vi "digitally_ros.vi"() -> ()   [LabVIEW 2019]
uses:
  <vilib>/addons/eal4LabVIEW/ApiLib/Connection control/ealApiConnect_string.vi
  <vilib>/addons/eal4LabVIEW/eal4LabVIEW.lvlib
panel:
  out "appended array":bool[](array[boolean])
  out "In Range? (1)":bool
  out "In Range? (2)":bool
  out "In Range? (3)":bool
  in  "condition 6":i32(ring) items=["AXIS_CONDITION_ACTIVE"=0, "AXIS_CONDITION_PARKING"=1, "AXIS_CONDITION_DEACTIVATED"=2, "AXIS_CONDITION_ACTIVE_DECOUPLED"=4, "AXIS_CONDITION_PARKING_DECOUPLED"=5, "AXIS_CONDITION_DEACTIVATED_DECOUPLED"=6, "AXIS_CONDITION_ACTIVE_PARAMETERIZATION"=8, "AXIS_CONDITION_PARKING_PARAMETERIZATION"=9, "AXIS_CONDITION_DEACTIVATED_PARAMETERIZATION"=10, "AXIS_CONDITION_ACTIVE_DECOUPLED_PARAMETERIZATION"=12, "AXIS_CONDITION_PARKING_DECOUPLED_PARAMETERIZATION"=13, "AXIS_CONDITION_DEACTIVATED_DECOUPLED_PARAMETERIZATION"=14]
  in  "slave index 6":i32
  in  "condition 5":i32(ring) items=["AXIS_CONDITION_ACTIVE"=0, "AXIS_CONDITION_PARKING"=1, "AXIS_CONDITION_DEACTIVATED"=2, "AXIS_CONDITION_ACTIVE_DECOUPLED"=4, "AXIS_CONDITION_PARKING_DECOUPLED"=5, "AXIS_CONDITION_DEACTIVATED_DECOUPLED"=6, "AXIS_CONDITION_ACTIVE_PARAMETERIZATION"=8, "AXIS_CONDITION_PARKING_PARAMETERIZATION"=9, "AXIS_CONDITION_DEACTIVATED_PARAMETERIZATION"=10, "AXIS_CONDITION_ACTIVE_DECOUPLED_PARAMETERIZATION"=12, "AXIS_CONDITION_PARKING_DECOUPLED_PARAMETERIZATION"=13, "AXIS_CONDITION_DEACTIVATED_DECOUPLED_PARAMETERIZATION"=14]
  in  "slave index 5":i32
  in  "condition 4":i32(ring) items=["AXIS_CONDITION_ACTIVE"=0, "AXIS_CONDITION_PARKING"=1, "AXIS_CONDITION_DEACTIVATED"=2, "AXIS_CONDITION_ACTIVE_DECOUPLED"=4, "AXIS_CONDITION_PARKING_DECOUPLED"=5, "AXIS_CONDITION_DEACTIVATED_DECOUPLED"=6, "AXIS_CONDITION_ACTIVE_PARAMETERIZATION"=8, "AXIS_CONDITION_PARKING_PARAMETERIZATION"=9, "AXIS_CONDITION_DEACTIVATED_PARAMETERIZATION"=10, "AXIS_CONDITION_ACTIVE_DECOUPLED_PARAMETERIZATION"=12, "AXIS_CONDITION_PARKING_DECOUPLED_PARAMETERIZATION"=13, "AXIS_CONDITION_DEACTIVATED_DECOUPLED_PARAMETERIZATION"=14]
  in  "slave index 4":i32
  out "RPM Motor 1":dbl
  out "RPM Motor 2":dbl
  out "RPM Motor 3":dbl
  in  "stop":bool
  out "return value":dbl[](array[numeric])
  out "Iteration counter":i32
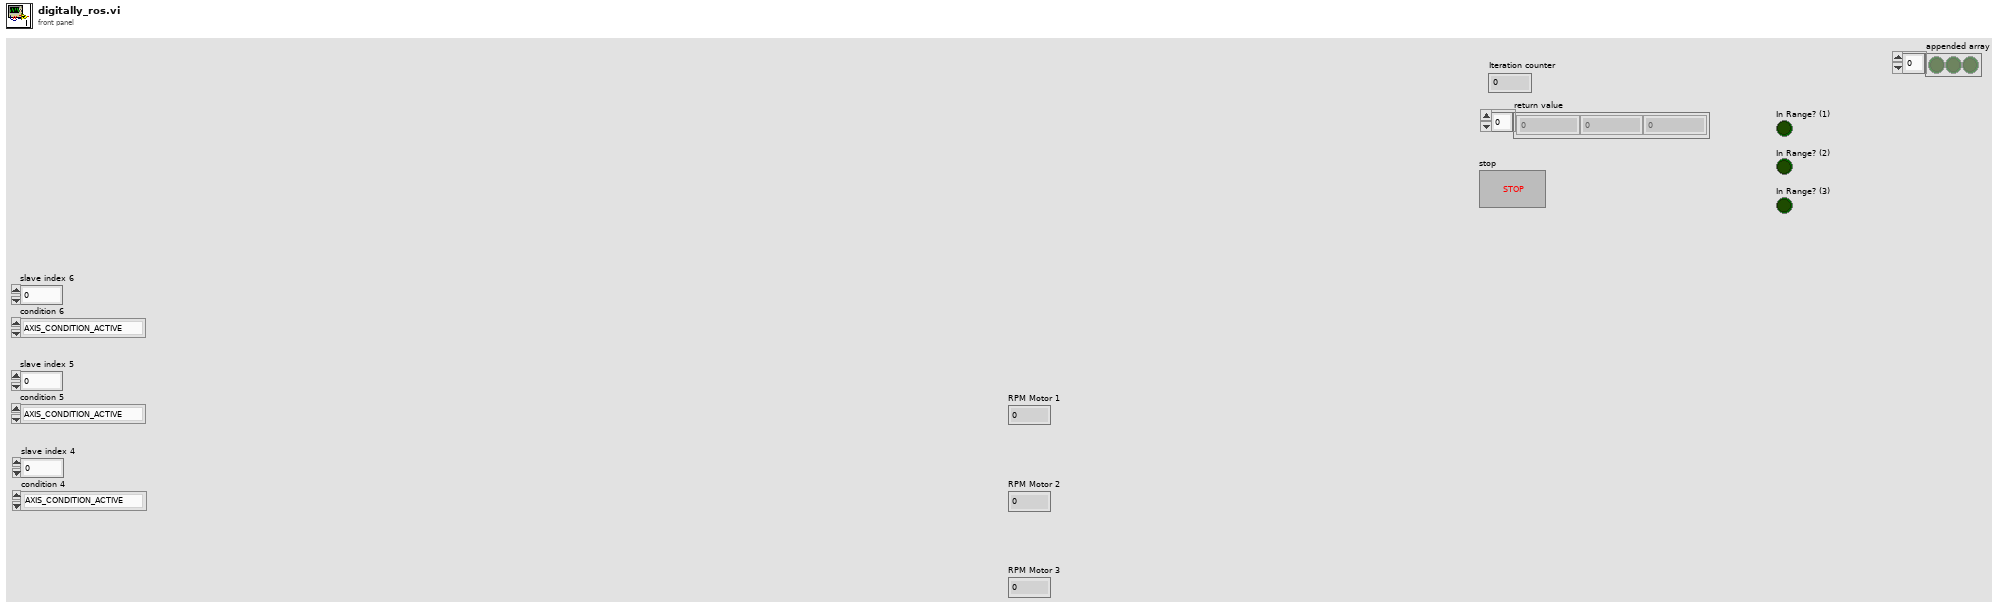
[diagram p1: front panel]
types:
  T1 = cluster{"Velocity":dbl, "Acceleration":dbl, "Deceleration":dbl, "Jerk":dbl}
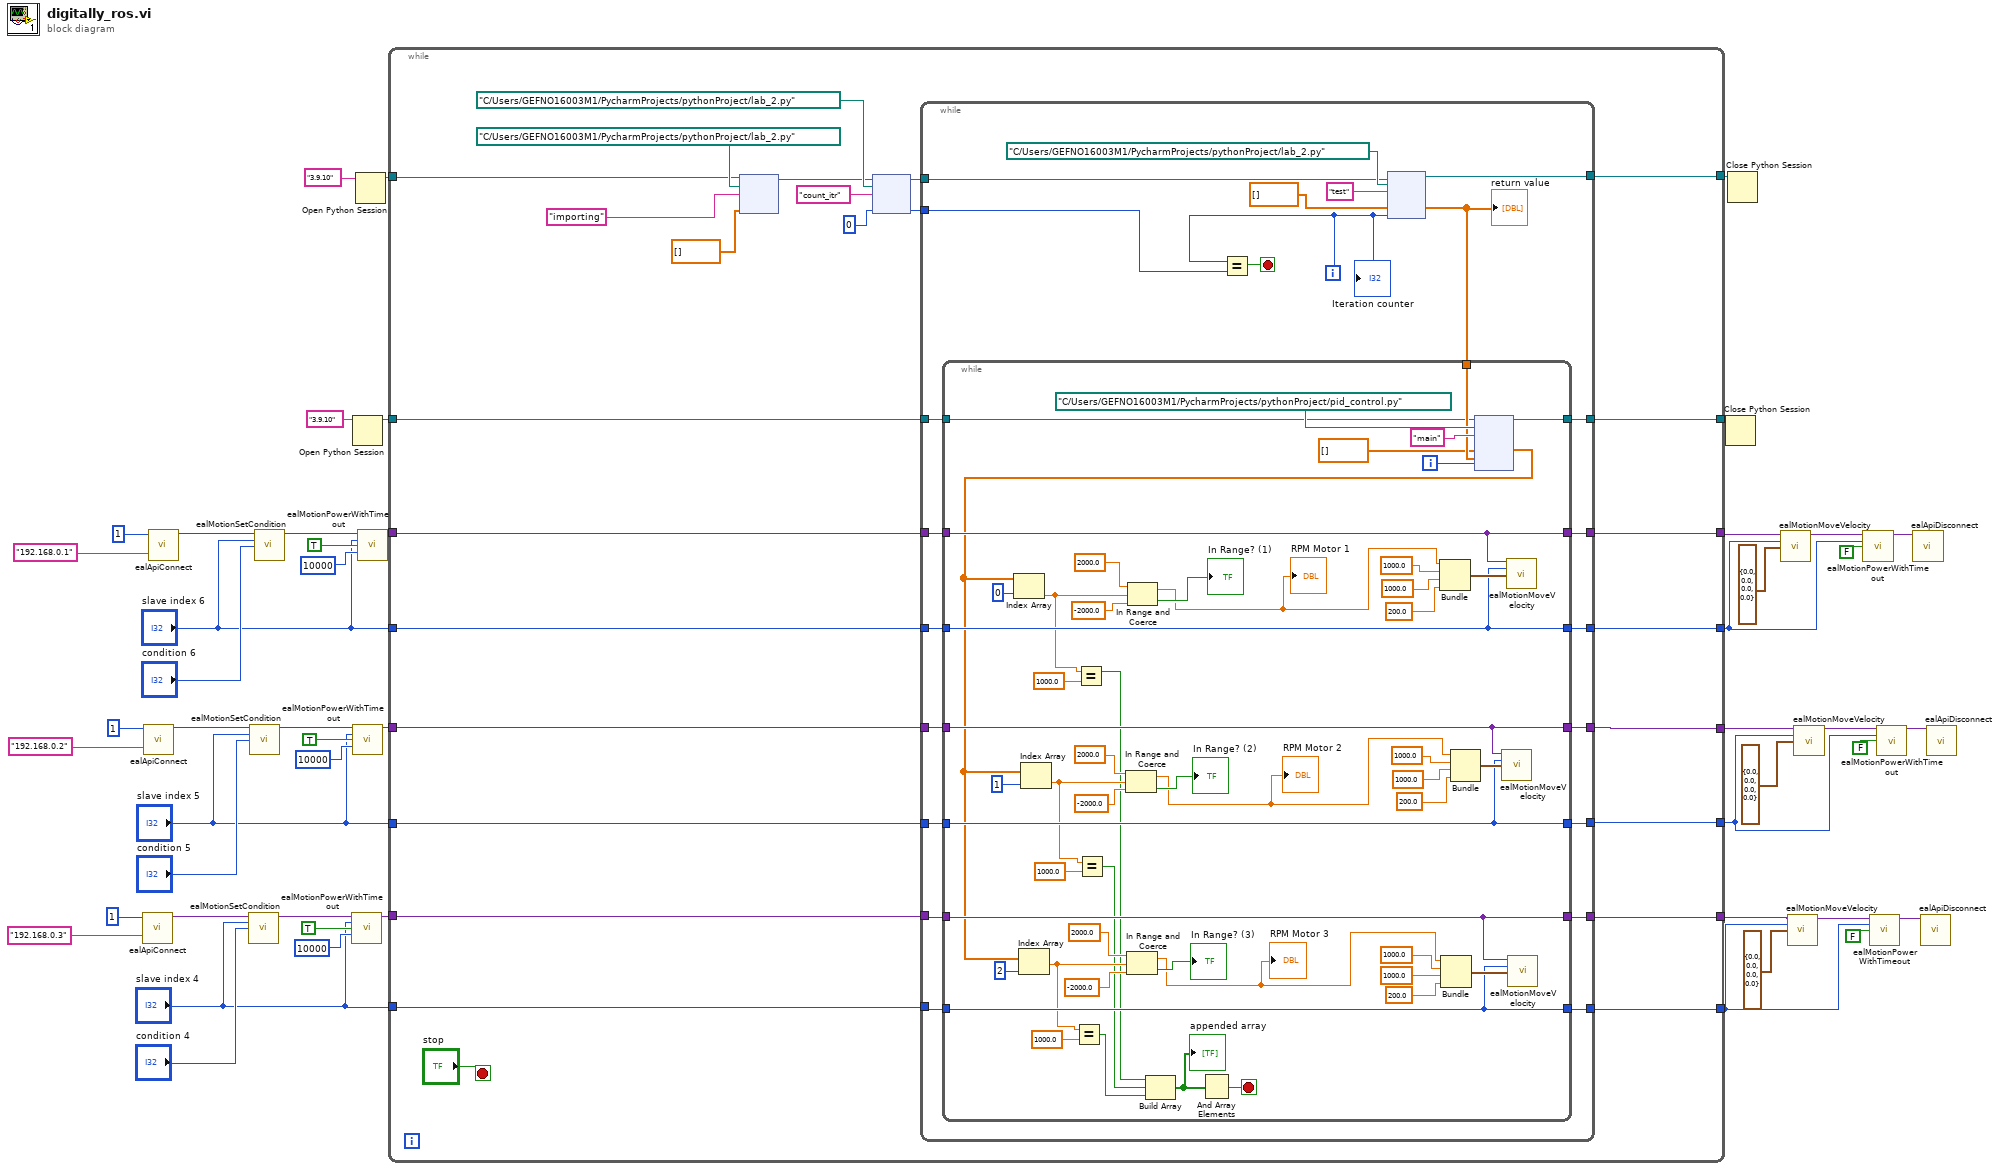
[diagram p0: block diagram]
diagram:
  n1 = call-poly <vilib>:"ealApiConnect.vi"("maximum no of axes"=1, "ip address"="192.168.0.3") -> ("connection out"=w37:variant)  [unwired: 12 in, 1 out]
  n2 = call-poly <vilib>:"ealApiConnect.vi"("maximum no of axes"=1, "ip address"="192.168.0.2") -> ("connection out"=w30:variant)  [unwired: 12 in, 1 out]
  n3 = call-poly <vilib>:"ealApiConnect.vi"("maximum no of axes"=1, "ip address"="192.168.0.1") -> ("connection out"=w23:variant)  [unwired: 12 in, 1 out]
  n4 = call <vilib>:"ealMotionSetCondition.vi"("connection in"=w37, "slave index"="slave index 4", "condition"="condition 4") -> ("connection out"=w36:variant)  [unwired: 11 in, 1 out]
  n5 = call <vilib>:"ealMotionSetCondition.vi"("connection in"=w30, "slave index"="slave index 5", "condition"="condition 5") -> ("connection out"=w29:variant)  [unwired: 11 in, 1 out]
  n6 = call <vilib>:"ealMotionSetCondition.vi"("connection in"=w23, "slave index"="slave index 6", "condition"="condition 6") -> ("connection out"=w22:variant)  [unwired: 11 in, 1 out]
  n7 = call <vilib>:"ealMotionPowerWithTimeout.vi"("connection in"=w36, "slave index"="slave index 4", "value"=TRUE, "timeout"=10000) -> ("connection out"=w16:variant)  [unwired: 10 in, 1 out]
  n8 = Open Python Session(python version="3.9.10" ("Python version")) -> (session out=w4:refnum<k35>)  [unwired: 2 in, 1 out]
  n9 = call <vilib>:"ealMotionPowerWithTimeout.vi"("connection in"=w29, "slave index"="slave index 5", "value"=TRUE, "timeout"=10000) -> ("connection out"=w17:variant)  [unwired: 10 in, 1 out]
  n10 = Open Python Session(python version="3.9.10" ("Python version")) -> (session out=w7:refnum<k35>)  [unwired: 2 in, 1 out]
  n11 = call <vilib>:"ealMotionPowerWithTimeout.vi"("connection in"=w22, "slave index"="slave index 6", "value"=TRUE, "timeout"=10000) -> ("connection out"=w18:variant)  [unwired: 10 in, 1 out]
  n12 = while {
    tunnel: w18 -> [w67]
    tunnel: w17 -> [w66]
    tunnel: w16 -> [w65]
    tunnel: [w64] -> w15
    tunnel: [w63] -> w14
    tunnel: "slave index 6" -> [w62]
    tunnel: "slave index 5" -> [w61]
    tunnel: [w60] -> w11
    tunnel: [w53] -> w10
    tunnel: "slave index 4" -> [w59]
    tunnel: w7 -> [w58]
    tunnel: [w57] -> w6
    tunnel: w4 -> [w56]
    tunnel: [w55] -> w3
    tunnel: [w54] -> w2
    tunnel: [w52] -> w1
    stop <- "stop" stop-if-true
    n13 = node(w58, path "C:/Users/GEFNO16003M1/PycharmProjects/pythonProject/lab_2.py" ("module path"), "importing" ("function name"), dbl[] []) -> (w72:refnum<k35>)  [unwired: 2 in, 3 out]
    n14 = node(w72, path "C:/Users/GEFNO16003M1/PycharmProjects/pythonProject/lab_2.py" ("module path"), "count_itr" ("function name"), 0) -> (w71:refnum<k35>, w69:i32)  [unwired: 1 in, 3 out]
    n15 = while {
      tunnel: [w94] -> w57
      tunnel: w71 -> [w97]
      tunnel: w69 -> [w95]
      tunnel: w67 -> [w92]
      tunnel: w66 -> [w81]
      tunnel: w65 -> [w91]
      tunnel: [w83] -> w64
      tunnel: [w84] -> w63
      tunnel: w62 -> [w82]
      tunnel: w61 -> [w80]
      tunnel: [w85] -> w60
      tunnel: w59 -> [w87]
      tunnel: w56 -> [w79]
      tunnel: [w89] -> w55
      tunnel: [w88] -> w54
      tunnel: [w86] -> w53
      tunnel: [w78] -> w52
      i -> [w90]
      stop <- w98 stop-if-true
      n16 = Equal?(x=w90, y=w95) -> (x = y?=w98:bool)
      n17 = node(w97, path "C:/Users/GEFNO16003M1/PycharmProjects/pythonProject/lab_2.py" ("module path"), "test" ("function name"), dbl[] [], w90) -> (w94:refnum<k35>, w93:dbl[])  [unwired: 2 in, 3 out]
      "return value" <- w93
      n18 = while {
        tunnel: w93 -> [w150]
        tunnel: w92 -> [w122]
        tunnel: w91 -> [w124]
        tunnel: [w124] -> w89
        tunnel: [w123] -> w88
        tunnel: w87 -> [w123]
        tunnel: [w120] -> w86
        tunnel: [w119] -> w85
        tunnel: [w121] -> w84
        tunnel: [w122] -> w83
        tunnel: w82 -> [w121]
        tunnel: w81 -> [w120]
        tunnel: w80 -> [w119]
        tunnel: w79 -> [w118]
        tunnel: [w117] -> w78
        i -> [w116]
        stop <- w114 stop-if-true
        n19 = node(w118, path "C:/Users/GEFNO16003M1/PycharmProjects/pythonProject/pid_control.py" ("module path"), "main" ("function name"), dbl[] [], w150, w116) -> (w117:refnum<k35>, w115:dbl[])  [unwired: 3 in, 3 out]
        n20 = Index Array(array=w115, index=0) -> (element=w110:dbl)
        n21 = Index Array(array=w115, index=2) -> (element=w108:dbl)
        n22 = Index Array(array=w115, index=1) -> (element=w109:dbl)
        n23 = Equal?(x=w108, y=1000.0) -> (x = y?=w105:bool)
        n24 = Equal?(x=w110, y=1000.0) -> (x = y?=w107:bool)
        n25 = Equal?(x=w109, y=1000.0) -> (x = y?=w106:bool)
        n26 = In Range and Coerce(upper limit=2000.0, x=w109, lower limit=-2000.0) -> (coerced(x)=w102:dbl, In Range?=→"In Range? (2)":bool)
        "RPM Motor 2" <- w102
        n27 = In Range and Coerce(upper limit=2000.0, x=w108, lower limit=-2000.0) -> (coerced(x)=w101:dbl, In Range?=→"In Range? (3)":bool)
        "RPM Motor 3" <- w101
        n28 = In Range and Coerce(upper limit=2000.0, x=w110, lower limit=-2000.0) -> (coerced(x)=w103:dbl, In Range?=→"In Range? (1)":bool)
        "RPM Motor 1" <- w103
        n29 = Build Array(w107, w106, w105) -> (w104:bool[])
        "appended array" <- w104
        n30 = And Array Elements(Boolean array=w104) -> (logical AND=w114:bool)
        n31 = Bundle("upper limit"=w103, 1000.0, 1000.0, 200.0) -> (w134:cluster{"upper limit":dbl, dbl, dbl, dbl})  [unwired: 1 in]
        n32 = Bundle("upper limit"=w101, 1000.0, 1000.0, 200.0) -> (w144:cluster{"upper limit":dbl, dbl, dbl, dbl})  [unwired: 1 in]
        n33 = Bundle("upper limit"=w102, 1000.0, 1000.0, 200.0) -> (w139:cluster{"upper limit":dbl, dbl, dbl, dbl})  [unwired: 1 in]
        n34 = call <vilib>:"ealMotionMoveVelocity.vi"("connection in"=w120, "slave index"=w119, "parameters set"=w139) -> ()  [unwired: 11 in, 2 out]
        n35 = call <vilib>:"ealMotionMoveVelocity.vi"("connection in"=w122, "slave index"=w121, "parameters set"=w134) -> ()  [unwired: 11 in, 2 out]
        n36 = call <vilib>:"ealMotionMoveVelocity.vi"("connection in"=w124, "slave index"=w123, "parameters set"=w144) -> ()  [unwired: 11 in, 2 out]
      }
      "Iteration counter" <- w90
    }
  }
  n37 = Close Python Session(session in=w1) -> ()  [unwired: 1 in, 1 out]
  n38 = Close Python Session(session in=w6) -> ()  [unwired: 1 in, 1 out]
  n39 = call <vilib>:"ealMotionMoveVelocity.vi"("connection in"=w15, "slave index"=w14, "parameters set"=T1 {"Velocity"=0.0, "Acceleration"=0.0, "Deceleration"=0.0, "Jerk"=0.0}) -> ("connection out"=w42:variant)  [unwired: 11 in, 1 out]
  n40 = call <vilib>:"ealMotionMoveVelocity.vi"("connection in"=w3, "slave index"=w2, "parameters set"=T1 {"Velocity"=0.0, "Acceleration"=0.0, "Deceleration"=0.0, "Jerk"=0.0}) -> ("connection out"=w50:variant)  [unwired: 11 in, 1 out]
  n41 = call <vilib>:"ealMotionMoveVelocity.vi"("connection in"=w10, "slave index"=w11, "parameters set"=T1 {"Velocity"=0.0, "Acceleration"=0.0, "Deceleration"=0.0, "Jerk"=0.0}) -> ("connection out"=w46:variant)  [unwired: 11 in, 1 out]
  n42 = call <vilib>:"ealMotionPowerWithTimeout.vi"("connection in"=w42, "slave index"=w14, "value"=FALSE) -> ("connection out"=w43:variant)  [unwired: 11 in, 1 out]
  n43 = call <vilib>:"ealMotionPowerWithTimeout.vi"("connection in"=w50, "slave index"=w2, "value"=FALSE) -> ("connection out"=w51:variant)  [unwired: 11 in, 1 out]
  n44 = call <vilib>:"ealMotionPowerWithTimeout.vi"("connection in"=w46, "slave index"=w11, "value"=FALSE) -> ("connection out"=w47:variant)  [unwired: 11 in, 1 out]
  n45 = call <vilib>:"ealApiDisconnect.vi"("connection in"=w43) -> ()  [unwired: 14 in, 1 out]
  n46 = call <vilib>:"ealApiDisconnect.vi"("connection in"=w51) -> ()  [unwired: 14 in, 1 out]
  n47 = call <vilib>:"ealApiDisconnect.vi"("connection in"=w47) -> ()  [unwired: 14 in, 1 out]
